vi "SUBVI Within Tolerance.vi"(8 "error in (no error)":errorcluster, 9 "Constant Value to Compare Against":dbl format="%0.2f", 10 "Tol":dbl=0.5 format="%0.4f", 11 "Operand 1":dynamicdata(graph)=[{"t0"=timestamp(0 s since 1904-01-01), "dt"=0.0001, "Y"=array[5000 elements], "attributes"=variant("NI_ChannelName"=variant(string "Sine"), "NI_ExpIsRelativeTime"=variant(bool TRUE), "NI_ExpStartTimeStamp"=variant(timestamp timestamp(3107453932.421 s since 1904-01-01)), "NI_ExpTimeStamp"=variant(timestamp timestamp(3107453932.421 s since 1904-01-01)), "NI_ExpXDimension"=variant(string "t"))}]) -> (0 "error out":errorcluster, 2 "Discrepancy":dbl, 3 "Result":dynamicdata(graph))   [LabVIEW 2018]
doc: "Compares input items you specify to determine whether values are equal, greater than, less than, and so on.\n--------------------\n\nThis Express VI is configured as follows:\n\nItems to Compare: Data points\nCompare Condition: = to within Tolerance\nTolerance: 0.5\nResults: One Result per Sample"
uses:
  <vilib>/express/express shared/comparison.ctl
panel:
  in  "Tab Control":enum32{"Page 1", "Page 2"}(tab)
  out "Signals In":dynamicdata(graph)=[{"t0"=timestamp(0 s since 1904-01-01), "dt"=0.0001, "Y"=array[5000 elements], "attributes"=variant("NI_ChannelName"=variant(string "Sine"), "NI_ExpIsRelativeTime"=variant(bool TRUE), "NI_ExpStartTimeStamp"=variant(timestamp timestamp(3107453932.421 s since 1904-01-01)), "NI_ExpTimeStamp"=variant(timestamp timestamp(3107453932.421 s since 1904-01-01)), "NI_ExpXDimension"=variant(string "t"))}]
  out "Signals In 2":dynamicdata(graph)=[{"t0"=timestamp(0 s since 1904-01-01), "dt"=0.0001, "Y"=array[5000 elements], "attributes"=variant("NI_ChannelName"=variant(string "Sine"), "NI_ExpIsRelativeTime"=variant(bool TRUE), "NI_ExpStartTimeStamp"=variant(timestamp timestamp(3107453992.3069997 s since 1904-01-01)), "NI_ExpTimeStamp"=variant(timestamp timestamp(3107453992.3069997 s since 1904-01-01)), "NI_ExpXDimension"=variant(string "t"))}]
  in  "Compare Condition":T1=enum."= to within Tolerance"
  in  "Invert Output":bool
  in  "Comparison Type":T2(ring)
  in  "Operand 2":dynamicdata(graph)=[{"t0"=timestamp(0 s since 1904-01-01), "dt"=0.0001, "Y"=array[5000 elements], "attributes"=variant("NI_ChannelName"=variant(string "Sine"), "NI_ExpIsRelativeTime"=variant(bool TRUE), "NI_ExpStartTimeStamp"=variant(timestamp timestamp(3107453992.3069997 s since 1904-01-01)), "NI_ExpTimeStamp"=variant(timestamp timestamp(3107453992.3069997 s since 1904-01-01)), "NI_ExpXDimension"=variant(string "t"))}]
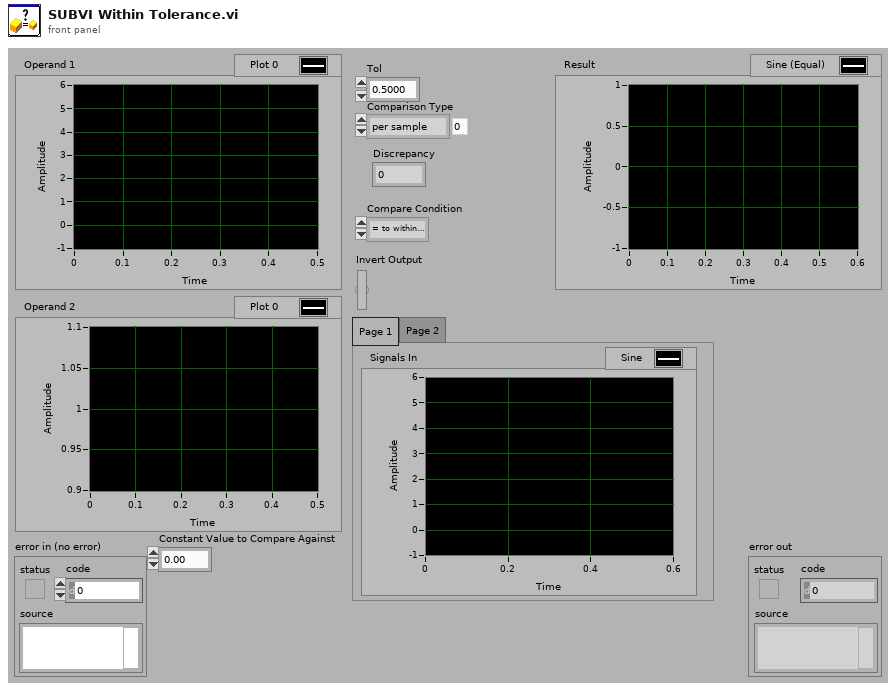
[diagram p1: front panel]
types:
  T1 = typedef "comparison.ctl" = enum16{"=", "Not Equal", ">", ">=", "<", "<=", "= to within Tolerance", "In Range", "Out of Range"}
  T2 = enum16{"per sample", "per channel", "all channels"}
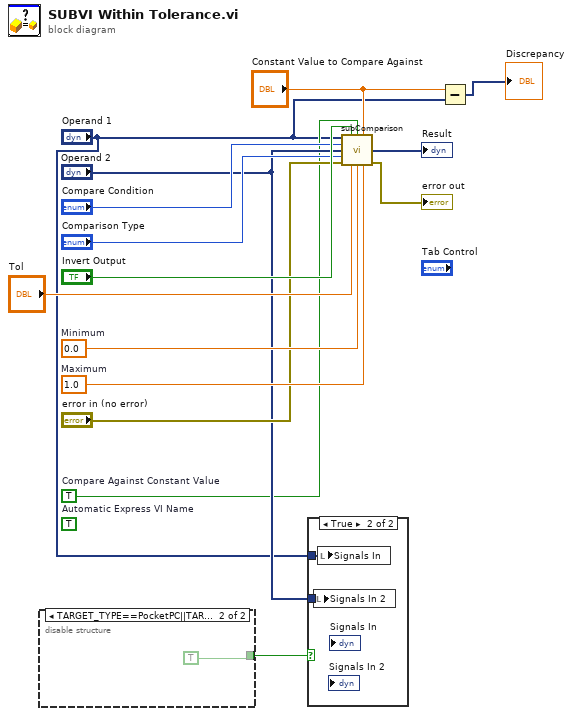
[diagram p0: block diagram]
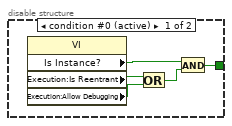
[diagram p2: hidden frame]
diagram:
  (unwired) TRUE  # Automatic Express VI Name
  w4 = TRUE  # Compare Against Constant Value
  w10 = 1.0  # Maximum
  w11 = 0.0  # Minimum
  n1 = disable-structure shown="TARGET_TYPE==PocketPC||TARGET_TYPE==PalmOS||TARGET_TYPE==Embedded" {
    disable-tunnel: [w20 TRUE] -> w6
    frame condition #0 (active) {
      n2 = property class="VI"() -> ("Is Instance?"=w19:bool, "Execution:Is Reentrant"=w17:bool, "Execution:Allow Debugging"=w16:bool)  [unwired: 2 in, 2 out]
      n3 = Or(x=w17, y=w16) -> (x .or. y?=w18:bool)
      n4 = And(x=w19, y=w18) -> (x .and. y?=w20:bool)
    }
    frame condition #1 {
    }
  }
  n5 = case shown="True" w6 {
    tunnel: "Operand 1" -> [_ w23]
    tunnel: "Operand 2" -> [_ w22]
    frame False {
    }
    frame True {
      n6 = local write "Signals In 2"(w22) -> ()
      n7 = local write "Signals In"(w23) -> ()
    }
  }
  n8 = call <vilib>:"subComparison.vi"("Input"="Operand 1", "Invert Output"="Invert Output", "Compare Against Constant Value"=w4, "Constant Value to Compare Against"="Constant Value to Compare Against", "Compare Condition"="Compare Condition", "Input 2"="Operand 2", "Comparison Type"="Comparison Type", "error in (no error)"="error in (no error)", "Tolerance"="Tol", "Minimum"=w11, "Maximum"=w10) -> ("Result"=→"Result":dynamicdata, "error out"=→"error out":errorcluster)  [unwired: 3 in]
  n9 = Subtract(x="Constant Value to Compare Against", y="Operand 1") -> (x-y=→"Discrepancy":dynamicdata)
